vi "Stop Counter.vi"() -> (0 "Error":errorcluster)   [LabVIEW 2011]
panel:
  # "by Paul Nathan, 01/03/2012"
  # "Revisions:\nDate       Desc.      Auth.\nx               x               x"
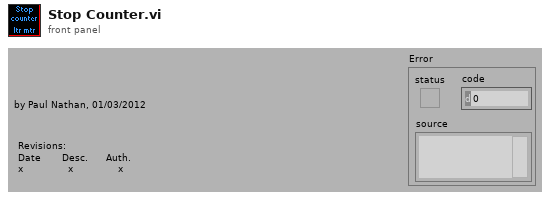
[diagram p1: front panel]
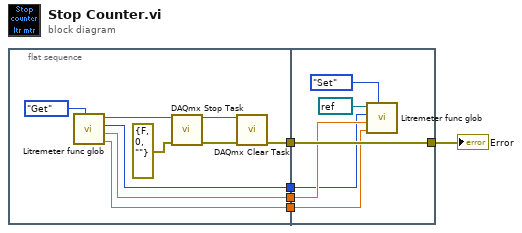
[diagram p0: block diagram]
diagram:
  n1 = flat-sequence {
    tunnel: [w11] -> w4
    tunnel: [w8] -> w3
    tunnel: [w7] -> w2
    tunnel: [w6] -> w1
    tunnel: [w20] -> w5
    tunnel: w4 -> [w20]
    tunnel: w3 -> [w17]
    tunnel: w2 -> [w16]
    tunnel: w1 -> [w15]
    frame #0 {
      n2 = call "Litremeter func glob.vi"("Action"=enum16{"Get", "Set"}."Get") -> ("Offset Litres out"=w8:dbl, "Litres / pulse out"=w7:dbl, "Pulse count out"=w6:u32, "Counter task out"=w9:refnum<k21>)  [unwired: 4 in, 1 out]
      n3 = call <vilib>:"DAQmx Stop Task.vi"("task/channels in"=w9, "error in"=errorcluster {"status"=FALSE, "code"=0, "source"=""}) -> ("task out"=w13:refnum<k21>, "error out"=w14:errorcluster)  [unwired: 12 in]
      n4 = call <vilib>:"DAQmx Clear Task.vi"("task in"=w13, "error in"=w14) -> ("error out"=w11:errorcluster)  [unwired: 13 in]
    }
    frame #1 {
      n5 = call "Litremeter func glob.vi"("Action"=enum16{"Get", "Set"}."Set", "Offset Litres in"=w17, "Litres / pulse in"=w16, "Pulse count in"=w15, "Counter task in"=refnum<k21> refnum) -> ()  [unwired: 5 out]
    }
  }
  "Error" <- w5
